vi "camera_synchrone_acquisition-ajg.vi"() -> ()   [LabVIEW 2020]
uses:
  <userlib>/WaveKit.lib/Controls/Image information.ctl
  <userlib>/WaveKit.lib/Controls/Image general information.ctl
  <userlib>/WaveKit.lib/Controls/Image acquisition information.ctl
  <userlib>/WaveKit.lib/Controls/Point2D.ctl
  <userlib>/WaveKit.lib/Controls/Data alignment enum.ctl
  <userlib>/WaveKit.lib/Classes/CameraSet/CameraSet.lvclass
  <userlib>/WaveKit.lib/Classes/Camera/Camera.lvclass
  <userlib>/WaveKit.lib/Classes/Image/Image.lvclass
panel:
  in  "Image in RAW":refnum<class "Image.lvclass">
  in  "Image in":refnum<class "Image.lvclass">
  in  "Camera.lvclass":refnum<class "Camera.lvclass">
  in  "CameraSet.lvclass":refnum<class "CameraSet.lvclass">
  out "Acquisition information":T1={"Image general information"={"Camera serial number"="", "Smearing removed"=FALSE, "Background image removed"=FALSE, "Time Stamp"=timestamp(0 s since 1904-01-01), "Comment"="", "Camera_MAX_Level"=0}, "Acquisition information"={"Exposure duration (us)"=0, "Exposure duration specified (us)"=0, "Gain"=0.0, "Number of summed images"=0, "Trigger type"=""}, "Number of pixels"={"X"=0, "Y"=0}, "Number of bits"=enum."16"}
  in  "Reset error":bool
  in  "acquisition_mode":enum16{"last_image", "new_image"}(ring)
  out "exposure_duration_us (get)":u32
  in  "exposure_duration_us (set)":u32=1000 min=1
  out "Current error":errorcluster
  in  "Exit":bool
  in  "Stop Acq":bool
  in  "Start Acq":bool
  out "Image Camera":u32[][](graph)
  in  "Configuration file path":path=path "C:/Program Files (x86)/Imagine Optic/Configuration Files/HASO4_first_7397.dat"
  # "Acquisition Parameters"
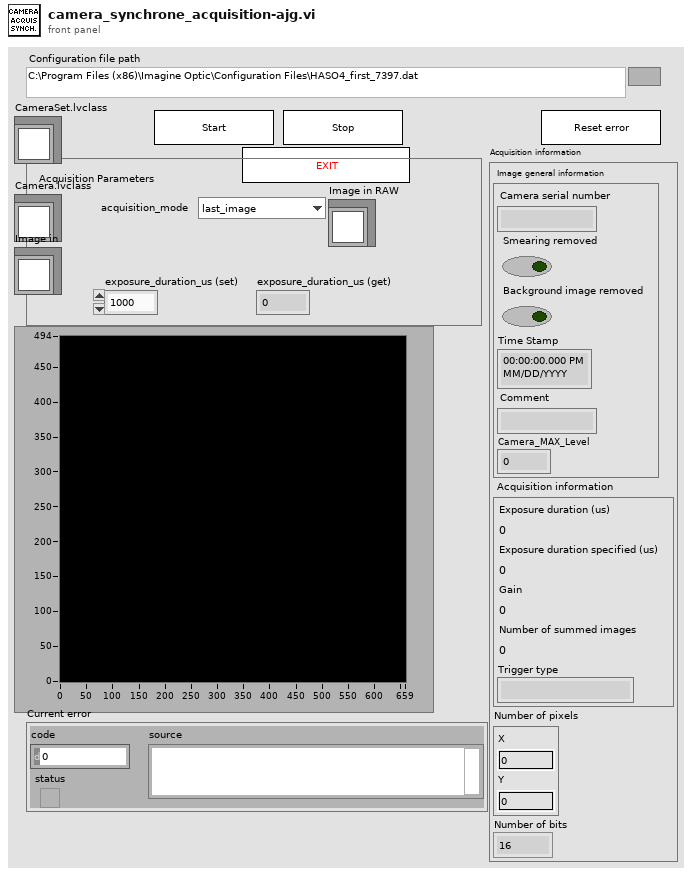
[diagram p1: front panel]
types:
  T1 = typedef "Image information.ctl" = cluster{"Image general information":T2, "Acquisition information":T3, "Number of pixels":T4, "Number of bits":T5}
  T2 = typedef "Image general information.ctl" = cluster{"Camera serial number":string, "Smearing removed":bool, "Background image removed":bool, "Time Stamp":timestamp, "Comment":string, "Camera_MAX_Level":i32}
  T3 = typedef "Image acquisition information.ctl" = cluster{"Exposure duration (us)":i32, "Exposure duration specified (us)":i32, "Gain":sgl, "Number of summed images":i32, "Trigger type":string}
  T4 = typedef "Point2D.ctl" = cluster{"X":u32, "Y":u32}
  T5 = typedef "Data alignment enum.ctl" = enum16{"8", "16", "32"}
  T6 = typedef "CameraSpecifications.ctl" = cluster{"Grabber name":string, "Camera name":string, "Camera sn":string, "Pixels_um":T7, "Maximum level":u32, "Data alignment":T5, "Is signed":bool, "Acquisition start":T4, "Acquisition length":T4, "MaxFrameRate_Hz":sgl, "Chip type":enum16{"Progressive scan", "Frame transfert"}}
  T7 = typedef "General dimensions definition.ctl" = cluster{"Size":T4, "Step":T8}
  T8 = typedef "Point2Df.ctl" = cluster{"X":sgl, "Y":sgl}
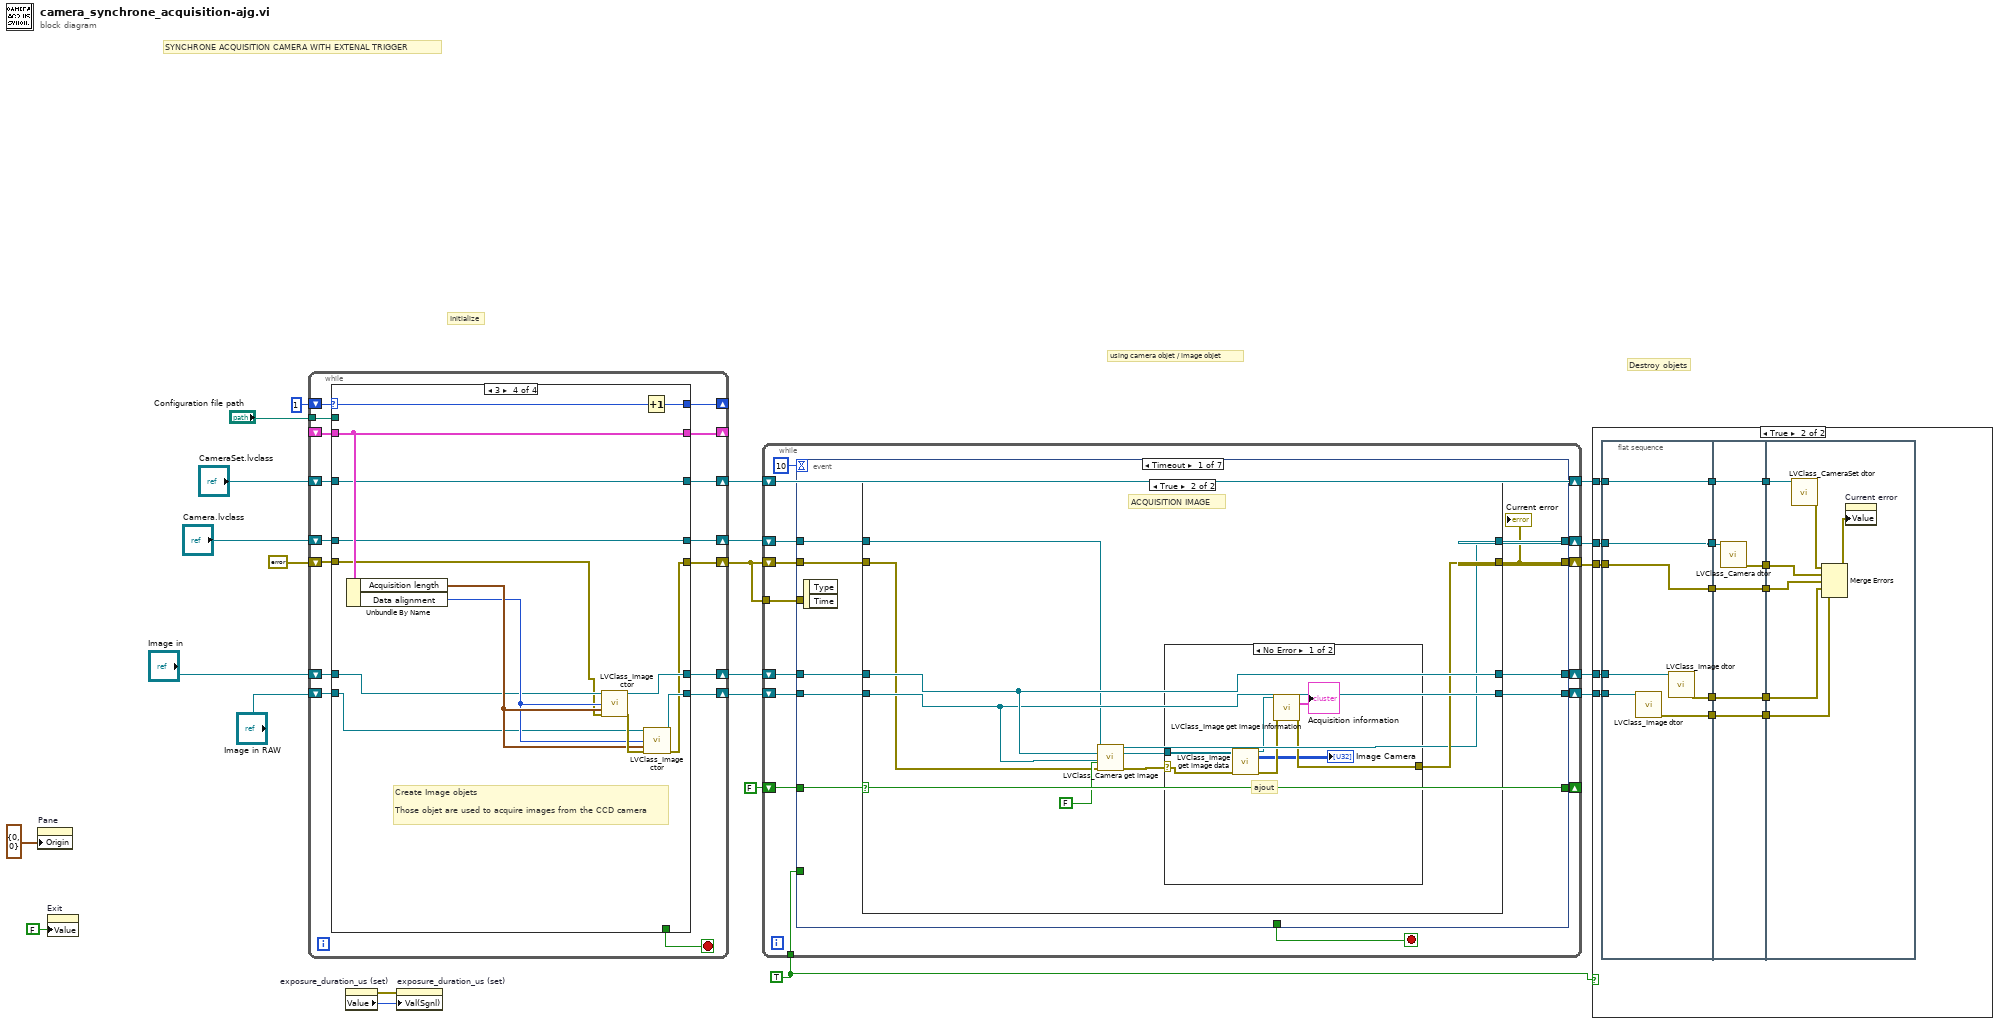
[diagram p0: block diagram]
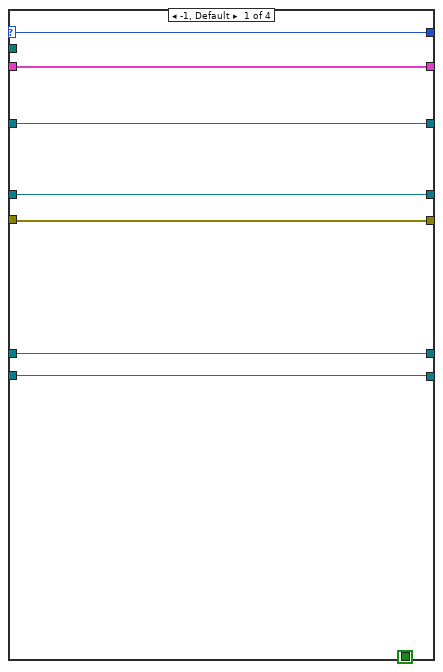
[diagram p2: hidden frame]
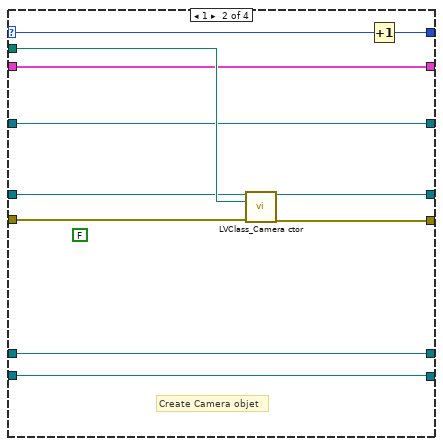
[diagram p3: hidden frame]
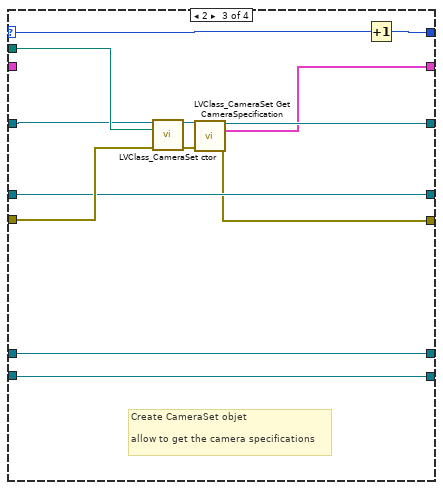
[diagram p4: hidden frame]
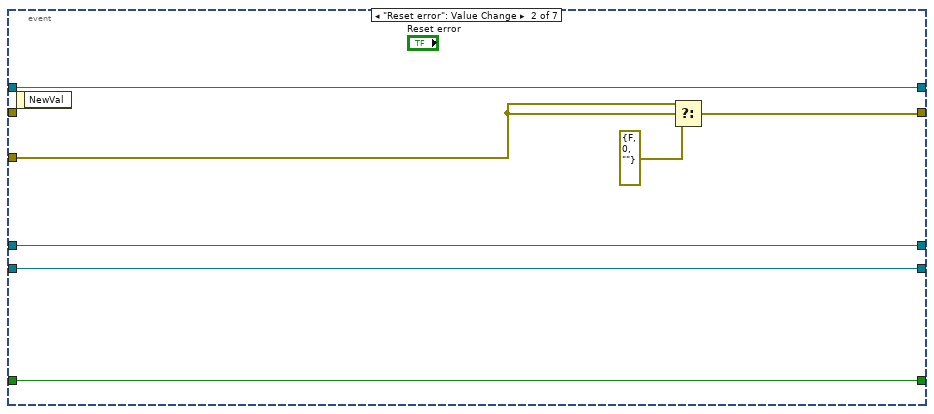
[diagram p8: hidden frame]
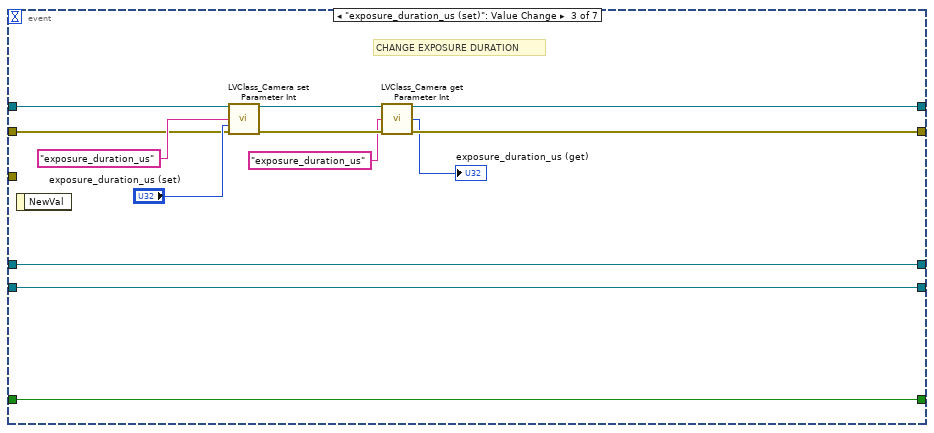
[diagram p9: hidden frame]
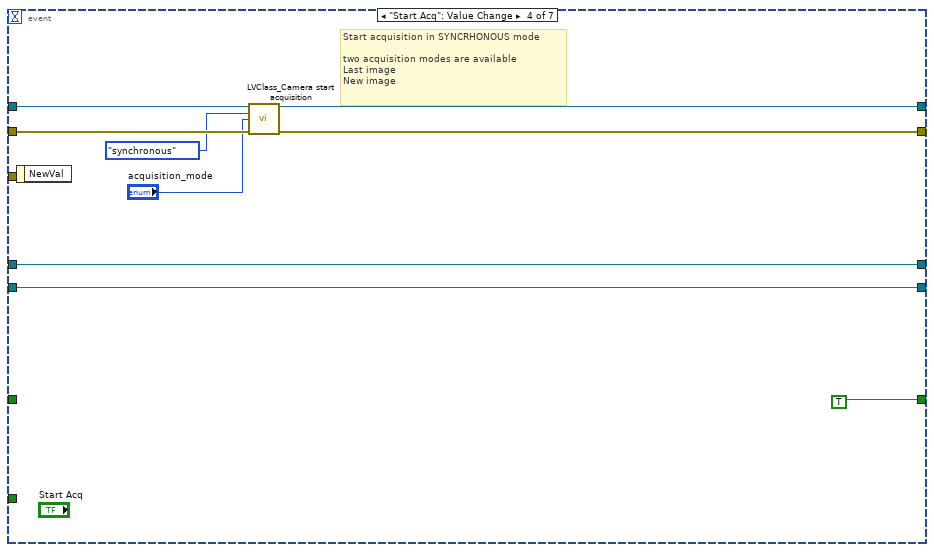
[diagram p10: hidden frame]
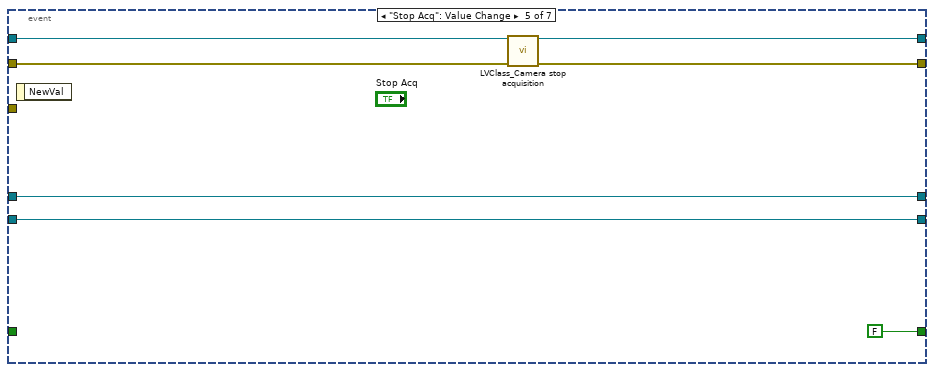
[diagram p11: hidden frame]
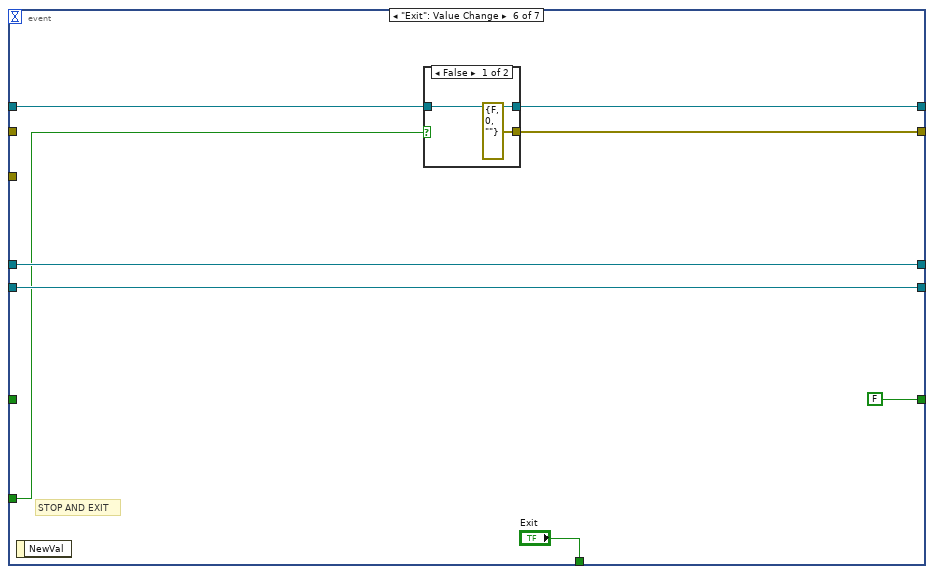
[diagram p12: hidden frame]
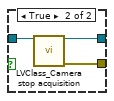
[diagram p13: hidden frame]
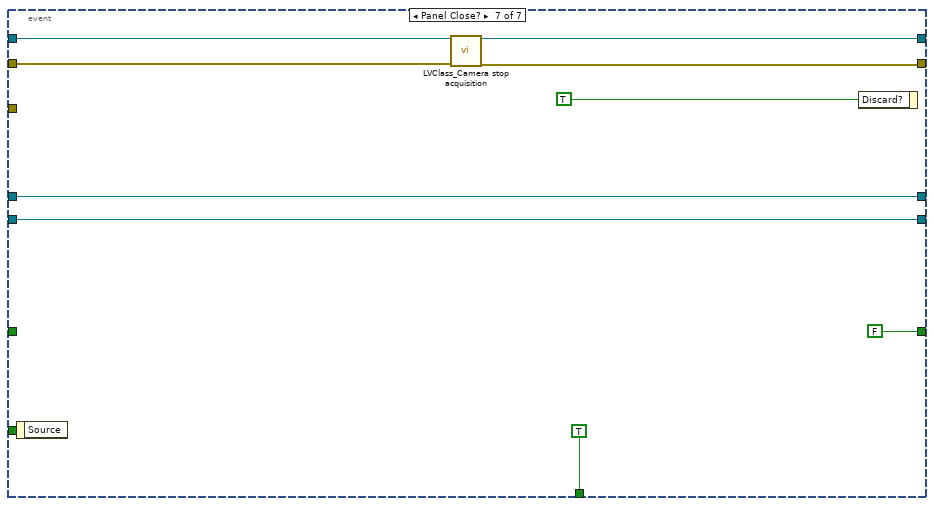
[diagram p14: hidden frame]
diagram:
  w7 = TRUE
  # "Destroy objets"
  # "using camera objet / image objet"
  # "Initialize"
  # "SYNCHRONE ACQUISITION CAMERA WITH EXTENAL TRIGGER"
  n1 = property on="Pane" class="Pane"("Origin"=cluster{"Horizontal":i16, "Vertical":i16} {"Horizontal"=0, "Vertical"=0} ("Front Panel Window:Origin")) -> ()  [unwired: 2 in, 2 out]
  n2 = property on="Exit" class="Bool (strict)"("Value"=FALSE ("Exit")) -> ()  [unwired: 2 in, 2 out]
  n3 = while {
    tunnel: "Configuration file path" -> [w37]
    shift-right: [w39] -> w17
    shift-left: "Camera.lvclass" -> [w33]
    shift-right: [w25] -> _
    shift-left: 1 -> [w24]
    shift-right: [w38] -> w16
    shift-left: "CameraSet.lvclass" -> [w32]
    shift-right: [w31] -> _
    shift-left: _ -> [w30]
    shift-right: [w36] -> w15
    shift-left: "Image in" -> [w28]
    shift-right: [w35] -> w14
    shift-left: "Image in RAW" -> [w29]
    shift-right: [w34] -> w8
    shift-left: errorcluster {"status"=FALSE, "code"=0, "source"=""} ("error out") -> [w26]
    stop <- w27 stop-if-true
    n4 = case shown="3" w24 {
      tunnel: [w47 w58 w64 w77] -> w39
      tunnel: w37 -> [_ w57 w68 _]
      tunnel: [w46 w55 w69 w78] -> w38
      tunnel: [w41 w51 w61 w82] -> w36
      tunnel: [w42 w52 w62 w81] -> w35
      tunnel: [w43 w54 w63 w80] -> w34
      selector: w24 -> [w40 w49 w60 w74]
      tunnel: w33 -> [w47 w56 w64 w77]
      tunnel: w32 -> [w46 w55 w67 w78]
      tunnel: [w44 w53 w66 w79] -> w31
      tunnel: w30 -> [w44 w53 _ w79]
      tunnel: w29 -> [w42 w52 w62 w76]
      tunnel: w28 -> [w41 w51 w61 w75]
      tunnel: [TRUE _ _ _] -> w27
      tunnel: w26 -> [w43 w48 w65 w72]
      tunnel: [w40 w50 w59 w73] -> w25
      frame -1, Default {
      }
      frame 1 {
        (unwired) FALSE ("Acq required")
        # "Create Camera objet"
        n5 = call <userlib>:"LVClass_Camera ctor.vi"("Camera"=w56, "Configuration file path"=w57, "error in (no error)"=w48) -> ("Camera (new)"=w58:refnum<class "Camera.lvclass">, "error out"=w54:errorcluster)  [unwired: 11 in]
        n6 = Increment(x=w49) -> (x+1=w50:i32)
      }
      frame 2 {
        # "Create CameraSet objet\n\nallow to get the camera specifications"
        n7 = call <userlib>:"LVClass_CameraSet ctor.vi"("CameraSet.lvclass"=w67, "Configuration file path"=w68, "error in (no error)"=w65) -> ("CameraSet.lvclass"=w71:refnum<class "CameraSet.lvclass">, "error out"=w70:errorcluster)  [unwired: 11 in]
        n8 = call <userlib>:"LVClass_CameraSet Get CameraSpecification.vi"("CameraSet.lvclass"=w71, "error in (no error)"=w70) -> ("CameraSet.lvclass"=w69:refnum<class "CameraSet.lvclass">, "Camera Config"=w66:T6, "error out"=w63:errorcluster)  [unwired: 11 in]
        n9 = Increment(x=w60) -> (x+1=w59:i32)
      }
      frame 3 {
        # "Create Image objets\n\nThose objet are used to acquire images from the CCD camera"
        n10 = Unbundle By Name(w79) -> ("Acquisition length"=w84:T4, "Data alignment"=w83:T5)
        n11 = call <userlib>:"LVClass_Image ctor.vi"("Image in"=w75, "Data alignment"=w83, "Size"=w84, "error in (no error)"=w72) -> ("Image out"=w82:refnum<class "Image.lvclass">, "error out"=w85:errorcluster)  [unwired: 10 in]
        n12 = Increment(x=w74) -> (x+1=w73:i32)
        n13 = call <userlib>:"LVClass_Image ctor.vi"("Image in"=w76, "Data alignment"=w83, "Size"=w84, "error in (no error)"=w85) -> ("Image out"=w81:refnum<class "Image.lvclass">, "error out"=w80:errorcluster)  [unwired: 10 in]
      }
    }
  }
  n14 = property on="exposure_duration_us (set)" class="DigNum (strict)"() -> (error out=w3:errorcluster, "Value"=w2:u32)  [unwired: 2 in, 1 out]
  n15 = property on="exposure_duration_us (set)" class="DigNum (strict)"(error in=w3, "Val(Sgnl)"=w2) -> ()  [unwired: 1 in, 2 out]
  n16 = while {
    shift-right: [w97] -> w23
    shift-left: w8 -> [w99]
    shift-right: [w95] -> w22
    shift-left: w17 -> [w96]
    shift-right: [w91] -> w21
    shift-left: w15 -> [w94]
    shift-right: [w90] -> w20
    shift-left: w14 -> [w93]
    shift-right: [w89] -> _
    shift-left: FALSE -> [w92]
    shift-right: [w88] -> w19
    shift-left: w16 -> [w88]
    tunnel: w8 -> [w87]
    tunnel: w7 -> [w86]
    stop <- w98 stop-if-true
    n17 = event shown="[0] Timeout" {
      selector: _ -> [_ _ _ _ _ _ _]
      dyn-events: _ -> [_ _ _ _ _ _ _]
      timeout: 10 -> [_ _ _ _ _ _ _]
      tunnel: w99 -> [w105 _ w148 w158 w160 _ w181]
      tunnel: [_ _ _ _ _ "Exit" TRUE ("Exit")] -> w98
      tunnel: [w101 w132 w143 w156 w164 w172 w184] -> w97
      tunnel: w96 -> [w108 w134 w147 w159 w165 w173 w186]
      tunnel: [w107 w134 w144 w157 w166 w171 w185] -> w95
      tunnel: w94 -> [w109 w136 w139 w152 w162 w169 w182]
      tunnel: w93 -> [w106 w137 w140 w151 w163 w170 w183]
      tunnel: w92 -> [w102 w135 w138 _ _ _ _]
      tunnel: [w104 w136 w139 w152 w162 w169 w182] -> w91
      tunnel: [w103 w137 w140 w151 w163 w170 w183] -> w90
      tunnel: [w102 w135 w138 TRUE FALSE FALSE FALSE] -> w89
      tunnel: w87 -> [_ w131 _ _ _ _ _]
      tunnel: w86 -> [_ _ _ _ _ w167 _]
      event Timeout {
        n18 = event-data() -> ()  [unwired: 1 in, 2 out]
        n19 = case shown="True" w102 {
          tunnel: [w110 w119] -> w101
          tunnel: w109 -> [w113 w122]
          tunnel: w106 -> [w112 w121]
          tunnel: [w113 w122] -> w104
          tunnel: [w112 w121] -> w103
          tunnel: w108 -> [w111 w116]
          tunnel: [w111 w115] -> w107
          tunnel: w105 -> [w110 w114]
          frame False {
          }
          frame True {
            # "ACQUISITION IMAGE"
            n20 = call <userlib>:"LVClass_Camera get image.vi"("Camera in"=w116, "Image"=w122, "Image RAW"=w121, "remove_background"=FALSE, "error in (no error)"=w114) -> ("Camera out"=w115:refnum<class "Camera.lvclass">, "Image (dup)"=w120:refnum<class "Image.lvclass">, "error out"=w117:errorcluster)  [unwired: 7 in, 1 out]
            n21 = case shown="No Error" w117 {
              selector: w117 -> [w129 w130]
              tunnel: [w126 w130] -> w119
              tunnel: w120 -> [w125 _]
              frame No Error {
                # "ajout"
                n22 = call <userlib>:"LVClass_Image get image data.vi"("Image in"=w125, "error in (no error)"=w129) -> ("Image out"=w128:refnum<class "Image.lvclass">, "Image data out"=→"Image Camera":u32[][], "error out"=w127:errorcluster)  [unwired: 11 in]
                n23 = call <userlib>:"LVClass_Image get image information.vi"("Image in"=w128, "error in (no error)"=w127) -> ("Acquisition information"=→"Acquisition information":T1, "error out"=w126:errorcluster)  [unwired: 11 in, 1 out]
              }
              frame Error {
              }
            }
          }
        }
        "Current error" <- w101
      }
      event "Reset error": Value Change {
        n24 = event-data() -> ()  [unwired: 1 in, 1 out]
        n25 = Select(t=w131, s=w131, f=errorcluster {"status"=FALSE, "code"=0, "source"=""} ("error out")) -> (s? t:f=w132:errorcluster)
      }
      event "exposure_duration_us (set)": Value Change {
        # "CHANGE EXPOSURE DURATION"
        n26 = event-data() -> ()  [unwired: 1 in, 1 out]
        n27 = call <userlib>:"LVClass_Camera set Parameter Int.vi"("Camera in"=w147, "parameter_name"="exposure_duration_us", "value"="exposure_duration_us (set)", "error in (no error)"=w148) -> ("Camera out"=w146:refnum<class "Camera.lvclass">, "error out"=w145:errorcluster)  [unwired: 10 in]
        n28 = call <userlib>:"LVClass_Camera get Parameter Int.vi"("Camera in"=w146, "parameter_name"="exposure_duration_us", "error in (no error)"=w145) -> ("Camera out"=w144:refnum<class "Camera.lvclass">, "value"=→"exposure_duration_us (get)":i32, "error out"=w143:errorcluster)  [unwired: 10 in]
      }
      event "Start Acq": Value Change {
        # "Start acquisition in SYNCRHONOUS mode\n\ntwo acquisition modes are available\nLast image\nNew image"
        n29 = event-data() -> ()  [unwired: 1 in, 1 out]
        n30 = call <userlib>:"LVClass_Camera start acquisition.vi"("Camera in"=w159, "synchronisation_mode"=enum16{"synchronous", "asynchronous"}."synchronous", "acquisition_mode"="acquisition_mode", "error in (no error)"=w158) -> ("Camera out"=w157:refnum<class "Camera.lvclass">, "error out"=w156:errorcluster)  [unwired: 10 in]
      }
      event "Stop Acq": Value Change {
        n31 = event-data() -> ()  [unwired: 1 in, 1 out]
        n32 = call <userlib>:"LVClass_Camera stop acquisition.vi"("Camera in"=w165, "error in (no error)"=w160) -> ("Camera out"=w166:refnum<class "Camera.lvclass">, "error out"=w164:errorcluster)  [unwired: 12 in]
      }
      event "Exit": Value Change {
        # "STOP AND EXIT"
        n33 = event-data() -> ()  [unwired: 1 in, 1 out]
        n34 = case shown="False" w167 {
          tunnel: w173 -> [w176 w179]
          tunnel: [errorcluster {"status"=FALSE, "code"=0, "source"=""} ("error out") w178] -> w172
          tunnel: [w176 w177] -> w171
          frame False {
          }
          frame True {
            n35 = call <userlib>:"LVClass_Camera stop acquisition.vi"("Camera in"=w179) -> ("Camera out"=w177:refnum<class "Camera.lvclass">, "error out"=w178:errorcluster)  [unwired: 13 in]
          }
        }
      }
      event Panel Close? {
        n36 = event-data() -> ()  [unwired: 1 in, 1 out]
        n37 = call <userlib>:"LVClass_Camera stop acquisition.vi"("Camera in"=w186, "error in (no error)"=w181) -> ("Camera out"=w185:refnum<class "Camera.lvclass">, "error out"=w184:errorcluster)  [unwired: 12 in]
        n38 = event-data("Discard?"=TRUE) -> ()  [unwired: 1 in, 1 out]
      }
    }
  }
  n39 = case shown="True" w7 {
    tunnel: w23 -> [_ w193]
    tunnel: w22 -> [_ w192]
    tunnel: w21 -> [_ w191]
    tunnel: w20 -> [_ w190]
    tunnel: w19 -> [_ w189]
    frame False {
    }
    frame True {
      n40 = flat-sequence {
        tunnel: w192 -> [w210]
        tunnel: w193 -> [w208]
        tunnel: [w210] -> w203
        tunnel: w189 -> [w209]
        tunnel: [w209] -> w202
        tunnel: [w208] -> w201
        tunnel: w191 -> [w207]
        tunnel: w190 -> [w206]
        tunnel: [w205] -> w200
        tunnel: [w204] -> w199
        tunnel: w203 -> [w216]
        tunnel: w202 -> [w215]
        tunnel: w201 -> [w213]
        tunnel: [w215] -> w198
        tunnel: [w214] -> w197
        tunnel: [w213] -> w196
        tunnel: w200 -> [w212]
        tunnel: [w212] -> w195
        tunnel: w199 -> [w211]
        tunnel: [w211] -> w194
        tunnel: w198 -> [w223]
        tunnel: w197 -> [w221]
        tunnel: w196 -> [w220]
        tunnel: w195 -> [w219]
        tunnel: w194 -> [w218]
        frame #0 {
          n41 = call <userlib>:"LVClass_Image dtor.vi"("Image in"=w206) -> ("error out"=w204:errorcluster)  [unwired: 13 in, 1 out]
          n42 = call <userlib>:"LVClass_Image dtor.vi"("Image in"=w207) -> ("error out"=w205:errorcluster)  [unwired: 13 in, 1 out]
        }
        frame #1 {
          n43 = call <userlib>:"LVClass_Camera dtor.vi"("Camera in"=w216) -> ("error out"=w214:errorcluster)  [unwired: 13 in, 1 out]
        }
        frame #2 {
          n44 = call <userlib>:"LVClass_CameraSet dtor.vi"("CameraSet.lvclass"=w223) -> ("error out"=w222:errorcluster)  [unwired: 13 in, 1 out]
          n45 = Merge Errors(w222, w221, w220, w219, w218) -> (w217:errorcluster)
          n46 = property on="Current error" class="Clust (strict)"("Value"=w217) -> ()  [unwired: 2 in, 2 out]
        }
      }
    }
  }
